vi "ESC Flight Profile Initial Plugin.vi"() -> (5 "Plug in titles":string[](array[string]), 7 "Plug in values":string[](array[string]))   [LabVIEW 2022 SP3]
uses:
  Controls/Post_Process.ctl
  Controls/Setup.ctl
  Controls/User_Specific_mode.ctl
  Globals/Trav_pos_global.vi
  Globals/Meas_global.vi
panel:
  out "Profile Filename":path
  in  "Milliseconds between Rendezvous and Acquisition starting":u32
  out "Case Currently On":string
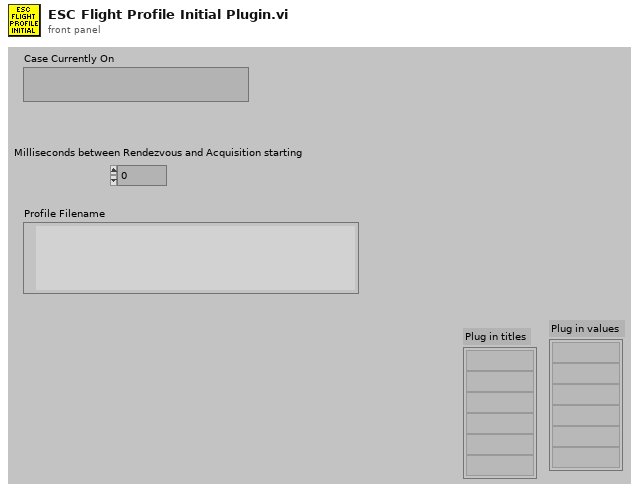
[diagram p1: front panel]
types:
  T1 = typedef "Traverse_cluster.ctl" = cluster{"Start X":sgl, "Start Y":sgl, "Start Z":sgl, "End X":sgl, "End Y":sgl, "End Z":sgl, "nPoints":i32, "Spacing":T2, "Filename":path, "Tunnel Speed":dbl, "Averaging time (mins)":dbl, "Extra Commands":string, "Carrier_1 Q (l/min)":dbl, "Carrier_2 Q (l/min)":dbl, "Trace Gas Concentration (%)":dbl, "Specific Arguments":string, "Comments":string, "Row No":i32, "Row Type Selector":T3, "EstCompl":string, "Row Duration (mins)":dbl, "nValidPoints":i32, "Meas Setup File":string}
  T2 = typedef "Spacing.ctl" = enum16{"Linear", "Log", "Gauss", "Specified", "N/A"}
  T3 = typedef "Multi_run_mode.ctl" = enum16{"Move Traverse Only", "Set Tunnel Speed Only", "Set Source Only", "Set Measurement Conditions", "Single Measurement", "Vertical Profile", "Lateral Profile", "Longitudinal Profile", "Multi-Axis Profile", "Explore Volume", "Auto Calibrate", "Meas Fast FID Bkgnd", "Check Beam Power", "Scanning Valve Measurement", "Run VI Named:", "Set ADAM Ch", "Wait (minutes)", "Send Message", "Synchronize With:", "Fall Back to this Row", "Turn Off Row Repeating", "Traverse 3D Volume", "Blank Row", "Jump to Fall Back Row"}
  T4 = typedef "Setup.ctl" = enum16{"Run Program", "Show Setup", "Save Current Setup", "Setup Front Panel"}
  T5 = typedef "Post_Process.ctl" = enum16{"Take New Data", "Post Process Raw Data File"}
  T6 = typedef "User_Specific_mode.ctl" = enum16{"Check VI only", "Run VI"}
  T7 = typedef "Rendezvous RefNum" = refnum<k1>
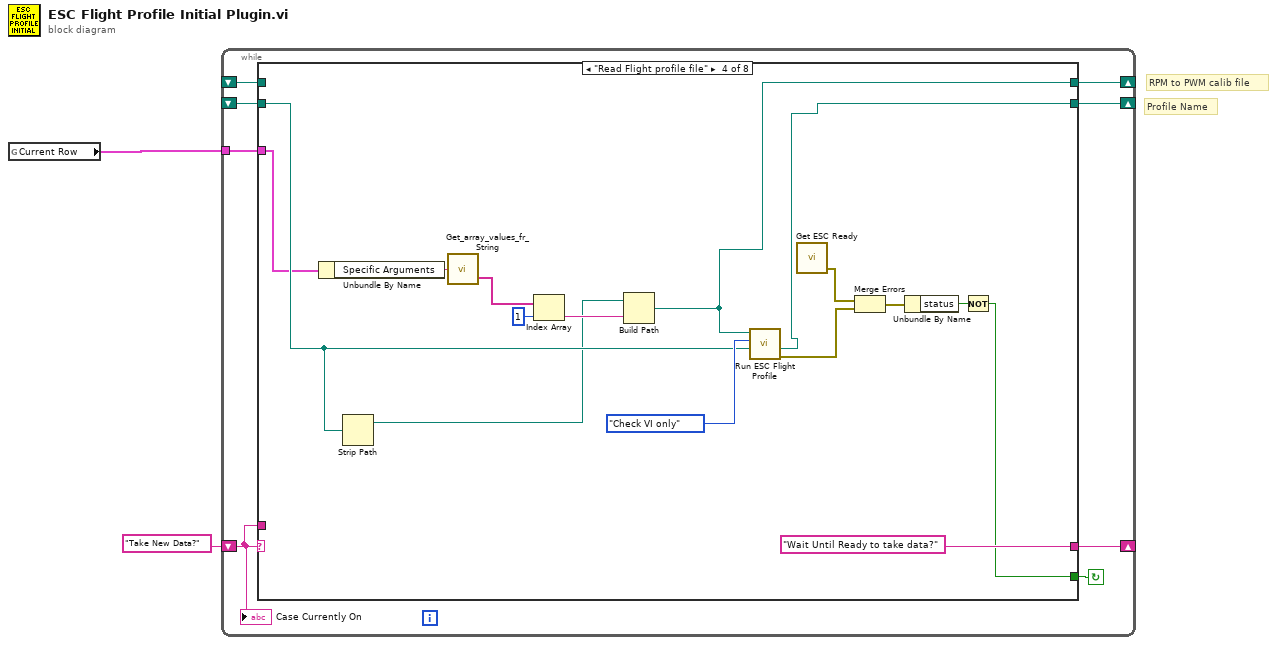
[diagram p0: block diagram]
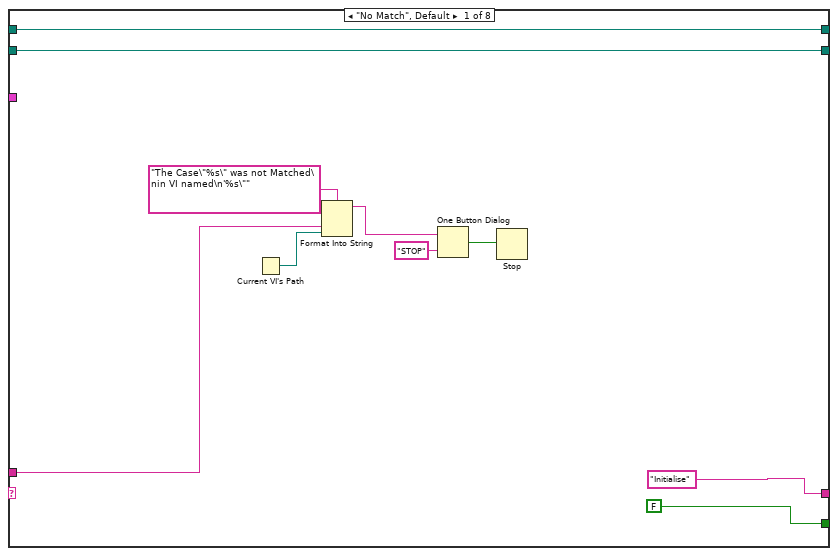
[diagram p2: hidden frame]
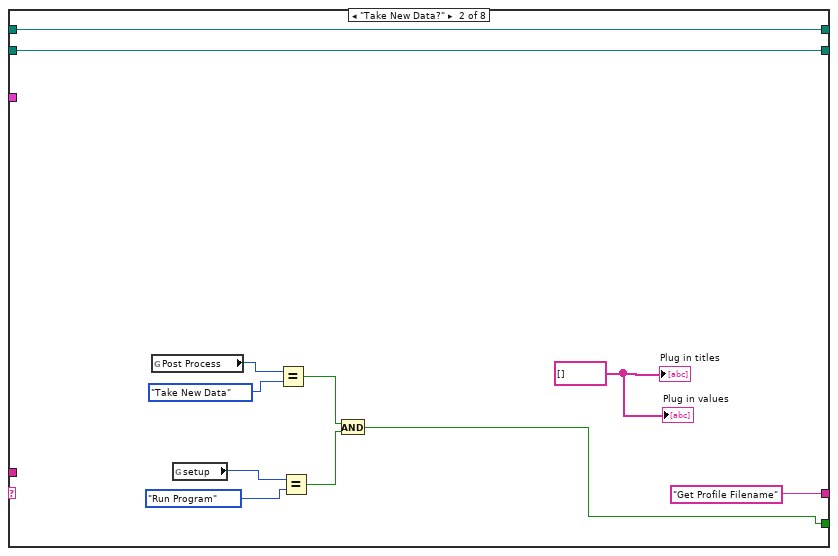
[diagram p3: hidden frame]
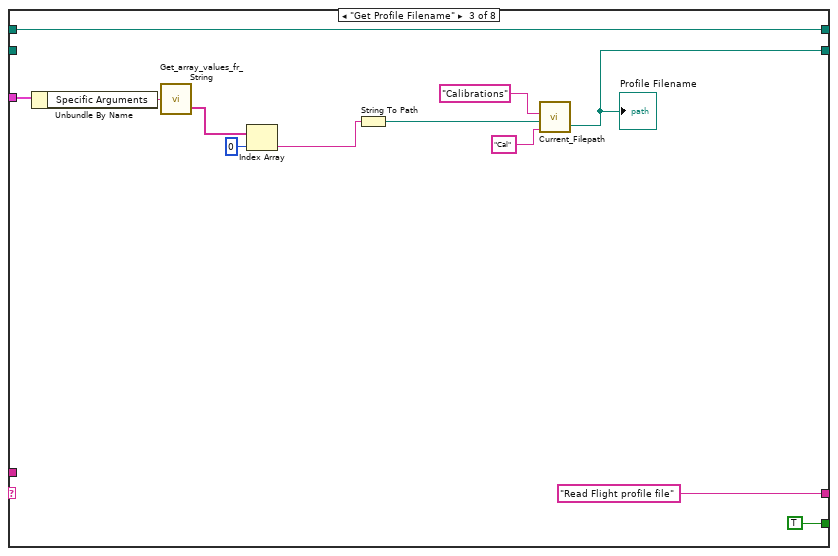
[diagram p4: hidden frame]
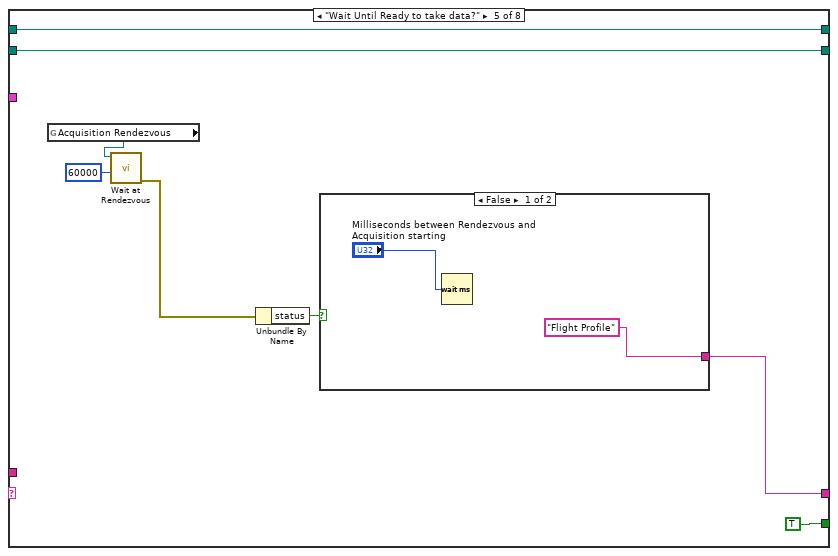
[diagram p5: hidden frame]
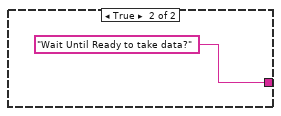
[diagram p6: hidden frame]
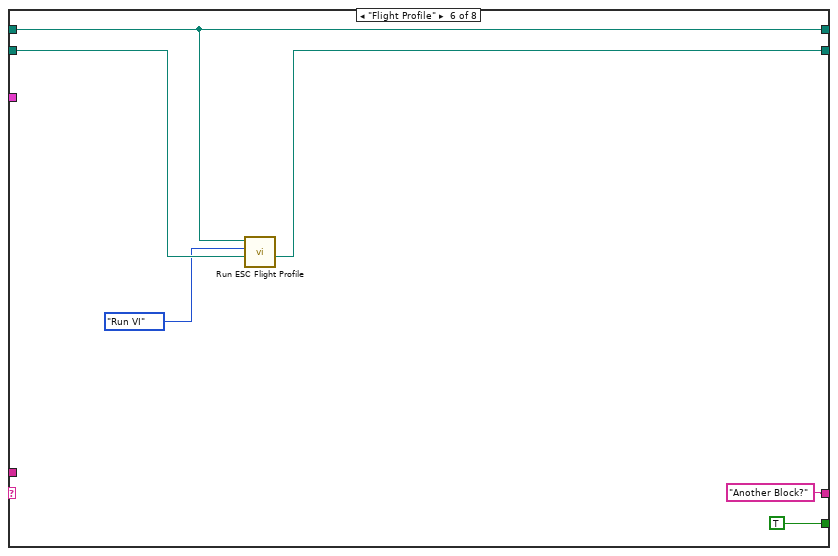
[diagram p7: hidden frame]
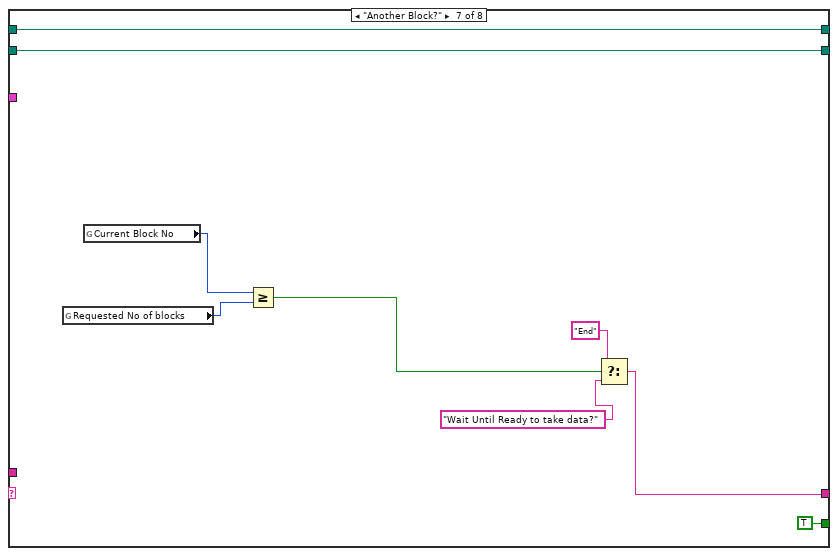
[diagram p8: hidden frame]
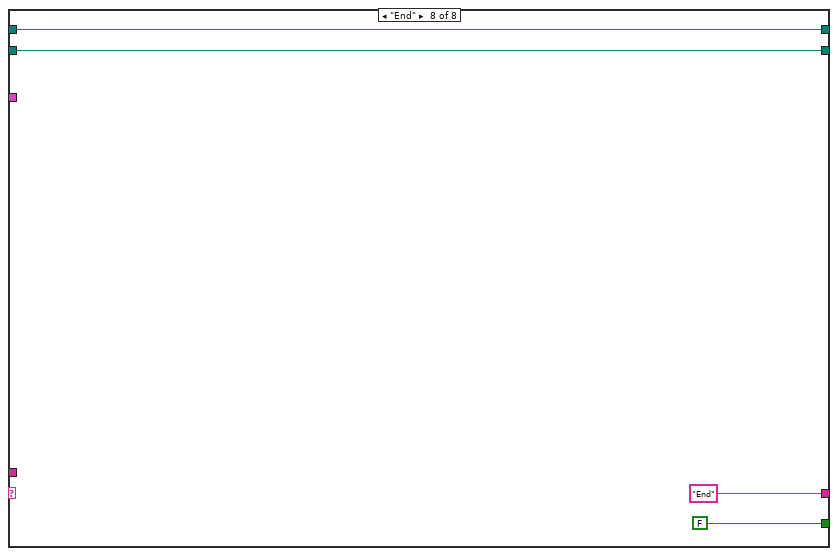
[diagram p9: hidden frame]
diagram:
  # "RPM to PWM calib file"
  # "Profile Name"
  n1 = global read "Trav_pos_global.vi" "Current Row"() -> (w1:T1)
  n2 = while {
    shift-left: "Take New Data?" -> [w8]
    shift-right: [w9] -> _
    tunnel: w1 -> [w7]
    shift-right: [w6] -> _
    shift-left: _ -> [w5]
    shift-right: [w4] -> _
    shift-left: _ -> [w3]
    stop <- w10 continue-if-true
    n3 = case shown="\"Read Flight profile file\"" w8 {
      tunnel: [FALSE w23 TRUE ("Command Found") w56 TRUE ("Command Found") TRUE ("Command Found") TRUE ("Command Found") FALSE ("Command Found")] -> w10
      tunnel: ["Initialise" "Get Profile Filename" "Read Flight profile file" ("f") "Wait Until Ready to take data?" ("f") w62 "Another Block?" w81 "End" ("f")] -> w9
      tunnel: w8 -> [w15 _ _ _ _ _ _ _]
      tunnel: w7 -> [_ _ w42 w48 _ _ _ _]
      tunnel: [w12 w22 w34 w52 w61 w71 w78 w87] -> w6
      tunnel: w5 -> [w12 w22 _ w51 w61 w74 w78 w87]
      tunnel: [w11 w21 w33 w44 w60 w72 w77 w86] -> w4
      tunnel: w3 -> [w11 w21 w33 _ w60 w72 w77 w86]
      frame "No Match", Default {
        n4 = Current VI's Path() -> (path=w14:path)
        n5 = Format Into String(format string="The Case\"%s\" was not Matched\nin VI named\n'%s\"" ("Format String"), w15, w14) -> (resulting string=w18:string)  [unwired: 2 in, 1 out]
        n6 = One Button Dialog(message=w18, button name ("OK")="STOP") -> (true=w16:bool)
        n7 = Stop(stop? (T)=w16) -> ()
      }
      frame "Take New Data?" {
        w28 = string[] [] ("Plug in titles")
        n8 = global read "Meas_global.vi" "Post Process"() -> (w30:T5)
        n9 = global read "Meas_global.vi" "setup"() -> (w27:T4)
        n10 = Equal?(x=w30, y=Post_Process."Take New Data" ("Post Process")) -> (x = y?=w24:bool)
        n11 = Equal?(x=w27, y=Setup."Run Program" ("setup")) -> (x = y?=w25:bool)
        n12 = And(x=w24, y=w25) -> (x .and. y?=w23:bool)
        "Plug in titles" <- w28
        "Plug in values" <- w28
      }
      frame "Get Profile Filename" {
        n13 = Unbundle By Name(w42) -> ("Specific Arguments"=w43:string)
        n14 = call "Get_array_values_fr_String.vi"("String Value"=w43) -> ("String array"=w41:string[])  [unwired: 1 out]
        n15 = Index Array(array=w41, index=0) -> (element=w36:string)
        n16 = String To Path(string=w36) -> (path=w35:path)
        n17 = call "Current_Filepath.vi"("Short_Name"="Cal" ("Data Type"), "Filename in"=w35, "Data Type"="Calibrations") -> ("Filename Out"=w34:path)  [unwired: 1 in, 1 out]
        "Profile Filename" <- w34
      }
      frame "Read Flight profile file" {
        n18 = Unbundle By Name(w48) -> ("Specific Arguments"=w50:string)
        n19 = Strip Path(path=w51) -> (stripped path=w45:path)  [unwired: 1 out]
        n20 = call "Get_array_values_fr_String.vi"("String Value"=w50) -> ("String array"=w49:string[])  [unwired: 1 out]
        n21 = Index Array(array=w49, index=1) -> (element=w46:string)
        n22 = Build Path(base path=w45, name or relative path=w46) -> (appended path=w44:path)
        n23 = call "Run ESC Flight Profile.vi"("Flight Profile File"=w51, "Simulate/Run"=User_Specific_mode."Check VI only", "RPM PWM Calib File"=w44) -> ("error IO"=w55:errorcluster, "Flight Profile Out"=w52:path)  [unwired: 7 in]
        n24 = call "Get ESC Ready.vi"() -> ("Error out"=w54:errorcluster)  [unwired: 4 in, 1 out]
        n25 = Merge Errors(w54, w55) -> (w53:errorcluster)
        n26 = Unbundle By Name(w53) -> ("status"=w57:bool)
        n27 = Not(x=w57) -> (.not. x?=w56:bool)
      }
      frame "Wait Until Ready to take data?" {
        n28 = global read "Meas_global.vi" "Acquisition Rendezvous"() -> (w65:T7)
        n29 = call <vilib>:"Wait at Rendezvous.vi"("ms timeout (-1)"=60000, "rendezvous"=w65) -> ("error out"=w64:errorcluster)  [unwired: 3 in, 2 out]
        n30 = Unbundle By Name(w64) -> ("status"=w63:bool)
        n31 = case shown="False" w63 {
          tunnel: ["Flight Profile" "Wait Until Ready to take data?" ("f")] -> w62
          frame False {
            n32 = Wait (ms)(milliseconds to wait="Milliseconds between Rendezvous and Acquisition starting") -> ()  [unwired: 1 out]
          }
          frame True {
          }
        }
      }
      frame "Flight Profile" {
        n33 = call "Run ESC Flight Profile.vi"("Flight Profile File"=w74, "Simulate/Run"=User_Specific_mode."Run VI", "RPM PWM Calib File"=w72) -> ("Flight Profile Out"=w71:path)  [unwired: 7 in, 1 out]
      }
      frame "Another Block?" {
        n34 = global read "Meas_global.vi" "Requested No of blocks"() -> (w85:i32)
        n35 = global read "Meas_global.vi" "Current Block No"() -> (w79:i32)
        n36 = Greater Or Equal?(x=w79, y=w85) -> (x >= y?=w83:bool)
        n37 = Select(t="End", s=w83, f="Wait Until Ready to take data?") -> (s? t:f=w81:string)
      }
      frame "End" {
      }
    }
    "Case Currently On" <- w8
  }
